vi "LVDimInterface.dim_operate.vi"(1 "DNSNode":string) -> ()   [LabVIEW 2012, in "LVDimInterface.lvlib"]
doc: "This VI should be started prior to any other VIs of the LVDimInterface. It should be kept running until LabVIEW is shut down.\n\nIt performs initialization of the DIM interface and ensures proper operation.\n\nHistory: 03-MAR-2006, Dietrich Beck\n\nCopyright (C)\nGesellschaft für Schwerionenforschung, GSI\nPlanckstr. 1\n64291 Darmstadt\nGermany\n\nContact: D.Beck@gsi.de \n\nThis program is free software; you can redistribute it and/or modify it under the terms of the \nGNU General Public License as published by the Free Software Foundation; either version 2 of the license, or (at your option) any later version.\n\nThis program is distributed in the hope that it will be useful, but WITHOUT ANY WARRANTY; without even the implied warranty of MERCHANTABILITY or FITNESS FOR A PARTICULAR PURPOSE. See the GNU General License for more details (http://www.gnu.org).\n\nGesellschaft für Schwerionenforschung, GSI\nPlanckstr. 1, 64291 Darmstadt, Germany\nFor all questions and ideas contact D. Beck.\nLast update: 16-DEC-2005"
uses:
  LVDimInterface.lvlib
  DimIndicators/DimIndicators.lvlib
  bin/libDimWrapper.so
panel:
  out "error out":errorcluster
  in  "stop":bool
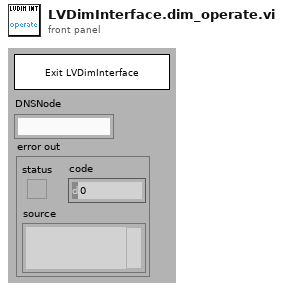
[diagram p1: front panel]
types:
  T1 = enum16{"unknown", "createSemaphore", "destroySemaphore", "getSemaphore"}
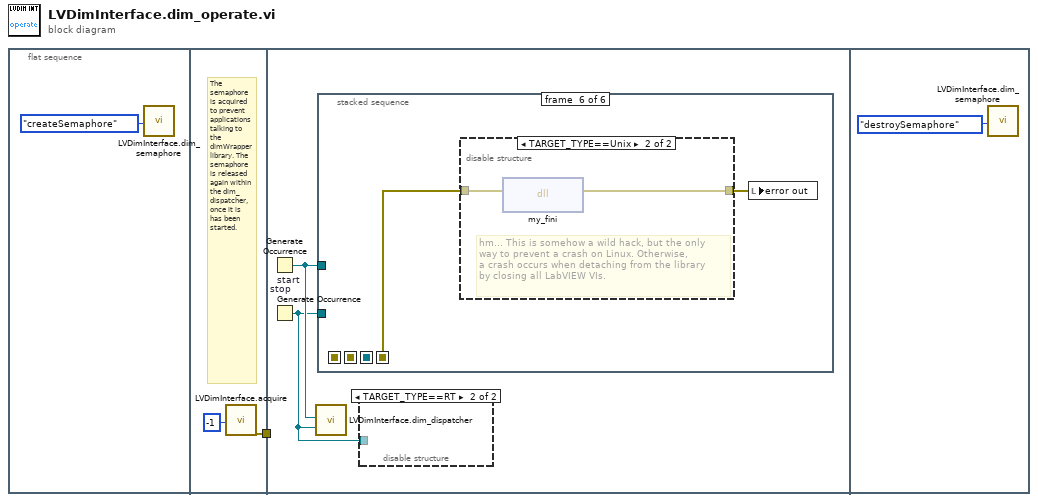
[diagram p0: block diagram]
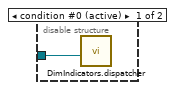
[diagram p2: hidden frame]
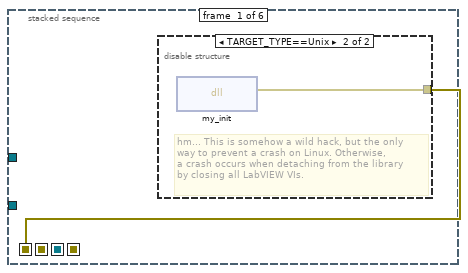
[diagram p3: hidden frame]
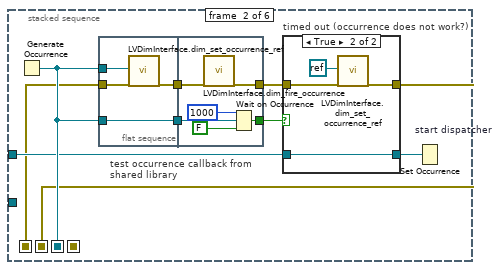
[diagram p5: hidden frame]
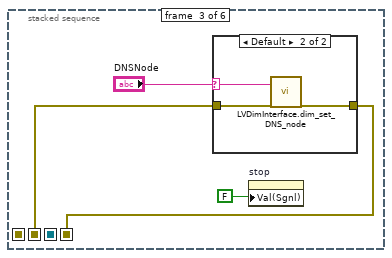
[diagram p7: hidden frame]
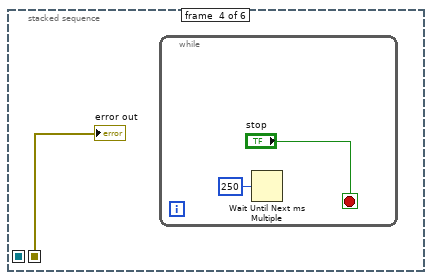
[diagram p9: hidden frame]
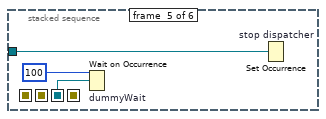
[diagram p10: hidden frame]
diagram:
  n1 = flat-sequence {
    tunnel: [w3] -> w1
    tunnel: w1 -> [_]
    frame #0 {
      n2 = call "LVDimInterface.dim_semaphore.vi"("Action"=T1."createSemaphore") -> ()  [unwired: 18 in, 1 out]
    }
    frame #1 {
      # "The semaphore is acquired to prevent applications talking to the dimWrapper library. The semaphore is released again within the dim_dispatcher, once it is has been started."
      n3 = call "LVDimInterface.acquire.vi"("ms timeout (10000)"=-1) -> ("error out"=w3:errorcluster)  [unwired: 17 in, 1 out]
    }
    frame #2 {
      n4 = Generate Occurrence "start"() -> (w6:refnum<k4>)
      n5 = Generate Occurrence "stop"() -> (w5:refnum<k4>)
      n6 = call "LVDimInterface.dim_dispatcher.vi"("start"=w6, "stop"=w5) -> ()  [unwired: 18 in]
      n7 = stacked-sequence {
        seq-local: [_ w18 _ _ _ _] -> [_ _ _ _ w48 _]
        seq-local: [w8 _ _ _ _ _] -> [_ w11 _ _ _ _]
        seq-local: [_ w10 _ _ _ _] -> [_ _ w36 _ _ _]
        seq-local: [_ _ w35 _ _ _] -> [_ _ _ w43 _ w50]
        tunnel: w6 -> [_ w17 _ _ _ _]
        tunnel: w5 -> [_ _ _ _ w46 _]
        frame #0 {
          n8 = disable-structure shown="TARGET_TYPE==Unix" {
            disable-tunnel: [_ w9] -> w8
            frame condition #0 (active) {
            }
            frame condition #1 {
              # "hm... This is somehow a wild hack, but the only\nway to prevent a crash on Linux. Otherwise,\na crash occurs when detaching from the library\nby closing all LabVIEW VIs."
              n9 = dll-call lib="D:/DIMLVEvent LV2012/bin/libDimWrapper.so" fn="my_init"() -> (error out=w9:errorcluster)  [unwired: 4 in, 1 out]
            }
          }
        }
        frame #1 {
          n10 = Generate Occurrence() -> (w18:refnum<k4>)
          n11 = flat-sequence "test occurrence callback from\nshared library" {
            tunnel: w18 -> [w22]
            tunnel: [w22] -> w15
            tunnel: w18 -> [w21]
            tunnel: [w20] -> w14
            tunnel: w11 -> [w19]
            tunnel: [w26] -> w13
            tunnel: [w25] -> w12
            tunnel: w15 -> [w28]
            tunnel: w14 -> [w24]
            frame #0 {
              n12 = call "LVDimInterface.dim_set_occurrence_ref.vi"("occurrence"=w21, "error in (no error)"=w19) -> ("error out"=w20:errorcluster)  [unwired: 17 in]
            }
            frame #1 {
              n13 = call "LVDimInterface.dim_fire_occurrence.vi"("error in (no error)"=w24) -> ("error out"=w25:errorcluster)  [unwired: 18 in]
              n14 = Wait on Occurrence(1:FALSE ("ignore previous (T)"), 2:w28, 3:1000 ("ms timeout (-1)")) -> (0:w26:bool)
            }
          }
          n15 = case "timed out (occurrence does not work?)" shown="True" w13 {
            tunnel: w12 -> [w29 w34]
            tunnel: w17 -> [w30 w32]
            tunnel: [w30 w32] -> w16
            tunnel: [w29 w31] -> w10
            frame False {
            }
            frame True {
              n16 = call "LVDimInterface.dim_set_occurrence_ref.vi"("occurrence"=refnum<k0> refnum ("Not a Refnum Constant"), "error in (no error)"=w34) -> ("error out"=w31:errorcluster)  [unwired: 17 in]
            }
          }
          n17 = Set Occurrence "start dispatcher"(w16) -> ()
        }
        frame #2 {
          n18 = case shown="Default" "DNSNode" {
            selector: "DNSNode" -> [_ w42]
            tunnel: w36 -> [w39 w41]
            tunnel: [w39 w40] -> w35
            frame "" {
            }
            frame Default {
              n19 = call "LVDimInterface.dim_set_DNS_node.vi"("DNS node"=w42, "error in (no error)"=w41) -> ("error out"=w40:errorcluster)  [unwired: 16 in, 1 out]
            }
          }
          n20 = property on="stop" class="Bool (strict)"("Val(Sgnl)"=FALSE ("Value (Signaling)")) -> ()  [unwired: 2 in, 2 out]
        }
        frame #3 {
          n21 = while {
            stop <- "stop" stop-if-true
            n22 = Wait Until Next ms Multiple(millisecond multiple=u32 250) -> ()  [unwired: 1 out]
          }
          "error out" <- w43
        }
        frame #4 {
          n23 = Wait on Occurrence "dummyWait"(2:w48, 3:100 ("ms timeout (-1)")) -> ()  [unwired: 1 in, 1 out]
          n24 = Set Occurrence "stop dispatcher"(w46) -> ()
        }
        frame #5 {
          n25 = disable-structure shown="TARGET_TYPE==Unix" {
            disable-tunnel: w50 -> [w51 w53]
            disable-tunnel: [w51 w52] -> w49
            frame condition #0 (active) {
            }
            frame condition #1 {
              # "hm... This is somehow a wild hack, but the only\nway to prevent a crash on Linux. Otherwise,\na crash occurs when detaching from the library\nby closing all LabVIEW VIs."
              n26 = dll-call lib="D:/DIMLVEvent LV2012/bin/libDimWrapper.so" fn="my_fini"(error in=w53) -> (error out=w52:errorcluster)  [unwired: 3 in, 1 out]
            }
          }
          n27 = local write "error out"(w49) -> ()
        }
      }
      n28 = disable-structure "Conditional Disable Structure" shown="TARGET_TYPE==RT" {
        disable-tunnel: w5 -> [w7 _]
        frame condition #0 (active) {
          n29 = call "DimIndicators.dispatcher.vi"("stop"=w7) -> ()  [unwired: 11 in]
        }
        frame condition #1 {
        }
      }
    }
    frame #3 {
      n30 = call "LVDimInterface.dim_semaphore.vi"("Action"=T1."destroySemaphore") -> ()  [unwired: 18 in, 1 out]
    }
  }
